vi "Read Passed count.vi"(11 "Test Suite Result In":T1) -> (2 "Pass count":i32, 3 "Test Suite Result Out":T1)   [LabVIEW 2020, in "Test Suite Result.lvlib"]
uses:
  Test Suite Result.lvlib
  Test Suite Result.ctl
  Assertion Result/Public/TypeDefs/Status.ctl
  Case Result/Test Case Result.ctl
  Method Result/Method Result.ctl
  Rewrite Project/Result/Status.ctl
  Assertion Result/Assertion Result.ctl
  Assertion Result/Public/TypeDefs/Assertion Type.ctl
  Case Result/Public/Read Status.vi
  Case Result/Private/Merge Status.vi
  Method Result/Public/Read Status.vi
  Assertion Result/Assertion Result.lvlib
  Method Result/Method Result.lvlib
  Case Result/Test Case Result.lvlib
  Rewrite Project/Result/Result.lvlib
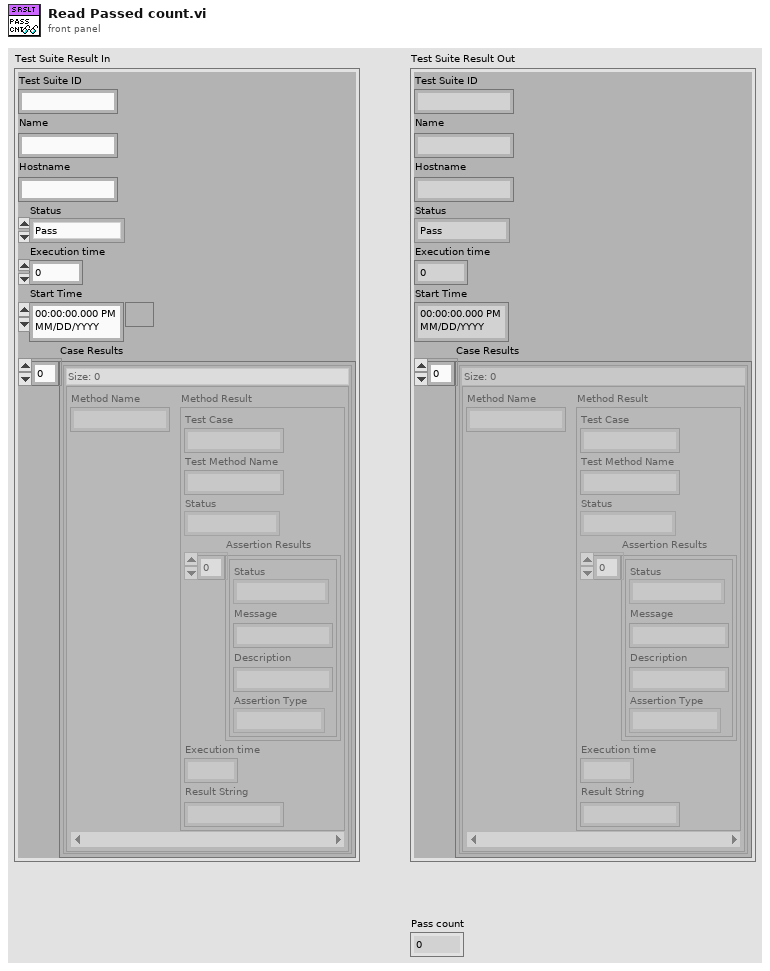
[diagram p1: front panel]
types:
  T1 = typedef "Test Suite Result.lvlib/Test Suite Result.ctl" = cluster{"Test Suite ID":string, "Name":string, "Hostname":string, "Status":T2, "Execution time":dbl, "Start Time":timestamp, "Case Results":T3[]}
  T2 = typedef "Assertion Result.lvlib/Status.ctl" = enum16{"Pass", "Fail", "Error", "Skipped", "Setup Error", "Broken", "Teardown Error"}
  T3 = typedef "Test Case Result.lvlib/Test Case Result.ctl" = map{string, T4}
  T4 = typedef "Method Result.lvlib/Method Result.ctl" = cluster{"Test Case":string, "Test Method Name":string, "Status":T5, "Assertion Results":T6[], "Execution time":dbl, "Result String":string}
  T5 = typedef "Result.lvlib/Status.ctl" = enum16{"Pass", "Fail", "Error", "Skipped", "Setup Error", "Broken", "Teardown Error"}
  T6 = typedef "Assertion Result.lvlib/Assertion Result.ctl" = cluster{"Status":T5, "Message":string, "Description":string, "Assertion Type":T7}
  T7 = typedef "Result.lvlib/Assertion Type.ctl" = enum16{"None", "Pass", "Fail", "Skip", "Pass if Equal", "Fail if Equal", "Pass if Error", "Fail if Error", "Pass if", "Fail if"}
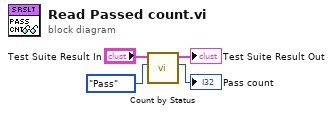
[diagram p0: block diagram]
diagram:
  n1 = call "Count by Status.vi"("Status"=Status."Pass", "Test Suite Result in"="Test Suite Result In") -> ("Count"=→"Pass count":i32, "Test Suite Result out"=→"Test Suite Result Out":T1)  [unwired: 8 in]
